vi "G#Debugger_RemoveObjectFromTree.vi"(0 "Front Panel":refnum<vi>, 1 "Tree":refnum<vi>, 2 "TreeElement":T1, 3 "hide empty classes?":bool, 5 "error in (no error)":errorcluster) -> (15 "EmptyTree?":bool, 19 "error out":errorcluster)   [LabVIEW 2017, in "G#Debugger.lvlib"]
uses:
  G#Debugger.lvlib
  G#Debugger_TreeElement.ctl
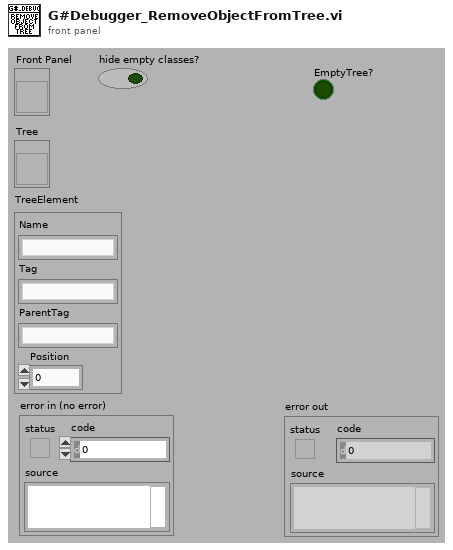
[diagram p1: front panel]
types:
  T1 = typedef "G#Debugger.lvlib/G#Debugger_TreeElement.ctl" = cluster{"Name":string, "Tag":string, "ParentTag":string, "Position":i32}
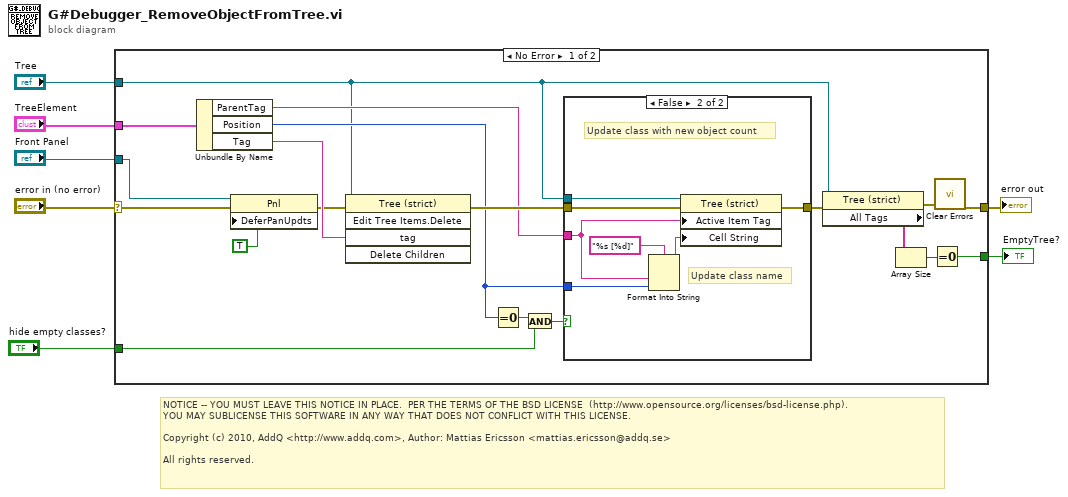
[diagram p0: block diagram]
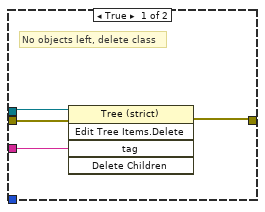
[diagram p2: hidden frame]
diagram:
  # "NOTICE -- YOU MUST LEAVE THIS NOTICE IN PLACE.  PER THE TERMS OF THE BSD LICENSE  (http://www.opensource.org/licenses/bsd-license.php).\nYOU MAY SUBLICENSE THIS SOFTWARE IN ANY WAY THAT DOES NOT CONFLICT WITH THIS LICENSE.\n\nCopyright (c) 2010, AddQ <http://www.addq.com>, Author: Mattias Ericsson <mattias.ericsson@addq.se>\n\nAll rights reserved."
  n1 = case shown="No Error" "error in (no error)" {
    selector: "error in (no error)" -> [w8 w38]
    tunnel: [w23 w38] -> w6
    tunnel: "Tree" -> [w16 _]
    tunnel: "TreeElement" -> [w26 _]
    tunnel: "hide empty classes?" -> [w19 _]
    tunnel: [w13 _] -> w2
    tunnel: "Front Panel" -> [w9 _]
    frame No Error {
      n2 = Unbundle By Name(w26) -> ("ParentTag"=w24:string, "Position"=w22:i32, "Tag"=w18:string)
      n3 = property class="Pnl"(reference=w9, error in=w8, "DeferPanUpdts"=TRUE ("Defer Panel Updates")) -> (error out=w12:errorcluster)  [unwired: 1 out]
      n4 = invoke class="Tree (strict)" method="Edit Tree Items.Delete"(reference=w16, error in=w12, "tag"=w18) -> (error out=w25:errorcluster)  [unwired: 2 in, 4 out]
      n5 = Equal To 0?(x=w22) -> (x = 0?=w20:bool)
      n6 = And(x=w20, y=w19) -> (x .and. y?=w21:bool)
      n7 = case shown="False" w21 {
        tunnel: w25 -> [w30 w37]
        tunnel: w16 -> [w29 w36]
        tunnel: [w28 w35] -> w17
        tunnel: w24 -> [w27 w34]
        tunnel: w22 -> [_ w31]
        frame True {
          # "No objects left, delete class"
          n8 = invoke class="Tree (strict)" method="Edit Tree Items.Delete"(reference=w29, error in=w30, "tag"=w27) -> (error out=w28:errorcluster)  [unwired: 2 in, 4 out]
        }
        frame False {
          # "Update class with new object count"
          # "Update class name"
          n9 = Format Into String(format string="%s [%d]", w34, w31) -> (resulting string=w32:string)  [unwired: 2 in, 1 out]
          n10 = property class="Tree (strict)"(reference=w36, error in=w37, "Active Item Tag"=w34, "Cell String"=w32) -> (error out=w35:errorcluster)  [unwired: 1 out]
        }
      }
      n11 = property class="Tree (strict)"(reference=w16, error in=w17) -> (error out=w10:errorcluster, "All Tags"=w15:string[])  [unwired: 1 out]
      n12 = Array Size(array=w15) -> (size(s)=w14:i32)
      n13 = Equal To 0?(x=w14) -> (x = 0?=w13:bool)
      n14 = call <vilib>:"Clear Errors.vi"("error in (no error)"=w10) -> ("error out"=w23:errorcluster)  [unwired: 5 in, 1 out]
    }
    frame Error {
    }
  }
  "error out" <- w6
  "EmptyTree?" <- w2
